vi "XY Graph Delete Consecutive Plots.vi"(8 "Error In":errorcluster, 9 "Plot Indices":i32[](array[numeric]), 11 "XY Graph Ref":refnum<vi>) -> (0 "Error Out":errorcluster, 1 "Plot Names":string[](array[string]), 2 "Graph Caption (or Label)":string, 3 "XY Graph Ref":refnum<vi>)   [LabVIEW 2021, in "XY Graph Add-Ons.lvlib"]
uses:
  XY Graph Add-Ons.lvlib
  Plot Update Steps.ctl
  XY Graph Plot Properties.ctl
  6eef607f-ca58-401d-bd43-5eec63f72193.vi
  XY Graph Get Plots Metadata.vi
  XY Graph Set Plots Metadata.vi
  Graphs.lvlib
  Arrays/Arrays.lvlib
  Error/Error.lvlib
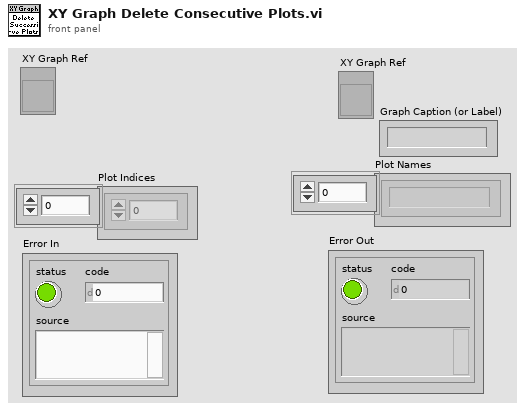
[diagram p1: front panel]
types:
  T1 = typedef "Graphs.lvlib/Plot Update Steps.ctl" = enum16{"Update Plot Styles", "Update Annotation List", "Update Cursor List", "Update Plots", "Quit"}
  T2 = typedef "XY Graph Add-Ons.lvlib/XY Graph Plot Properties.ctl" = cluster{"Plot Index":i32, "Plot.Bar Plot Style":u8, "Plot.DigitalLineStyle":u8, "Plot.TransitionLocation":u8, "Plot.Transition Type":u8, "Plot.Fill To":i16, "Plot.Fill/Pt. Color":u32, "Plot.Label Format":u8, "Plot.Line Style":u8, "Plot.Line Width":u8, "Plot.Plot Color":u32, "Plot.Plot Interpolation":u8, "Plot.Plot Name":string, "Plot.Point Style":u8, "Plot.Visible?":bool, "Plot.XScaleIdx":u32, "Plot.YScaleIdx":u32, "Plot.Anti-aliased":bool}
  T3 = typedef "LVAnnotationListTypeDef.ctl" = cluster{"Name":string, "Color":u32, "Style":u8, "Point Style":u8, "Name Visible":bool, "Allow Drag":bool, "Annotation Mode":u32, "Plot":i32, "Index":i32, "Position":cluster{"X":dbl, "Y":dbl}, "X Scale":u32, "Y Scale":u32, "Show Arrow":bool, "Lock Name":bool, "Plot Area":i32, "Label Offset":cluster{"X":dbl, "Y":dbl}}[]
  T4 = typedef "LVCursorListTypeDef.ctl" = cluster{"Name":string, "Color":u32, "Style":u8, "Point Style":u8, "Name Visible":bool, "Allow Drag":bool, "Cursor Mode":u32, "Plot":i32, "Index":i32, "Position":cluster{"X":dbl, "Y":dbl}, "X Scale":u32, "Y Scale":u32, "Watch Plots":i32[], "Watch All Plots":bool, "Plot Area":i32, "Label Offset":cluster{"X":dbl, "Y":dbl}}[]
  T5 = typedef "XY Graph Add-Ons.lvlib/XY Graph Refnum.ctl" = refnum<vi>
  T6 = cluster{"Name":string, "Color":u32, "Style":u8, "Point Style":u8, "Name Visible":bool, "Allow Drag":bool, "Annotation Mode":u32, "Plot":i32, "Index":i32, "Position":cluster{"X":dbl, "Y":dbl}, "X Scale":u32, "Y Scale":u32, "Show Arrow":bool, "Lock Name":bool, "Plot Area":i32, "Label Offset":cluster{"X":dbl, "Y":dbl}}
  T7 = cluster{"Name":string, "Color":u32, "Style":u8, "Point Style":u8, "Name Visible":bool, "Allow Drag":bool, "Cursor Mode":u32, "Plot":i32, "Index":i32, "Position":cluster{"X":dbl, "Y":dbl}, "X Scale":u32, "Y Scale":u32, "Watch Plots":i32[], "Watch All Plots":bool, "Plot Area":i32, "Label Offset":cluster{"X":dbl, "Y":dbl}}
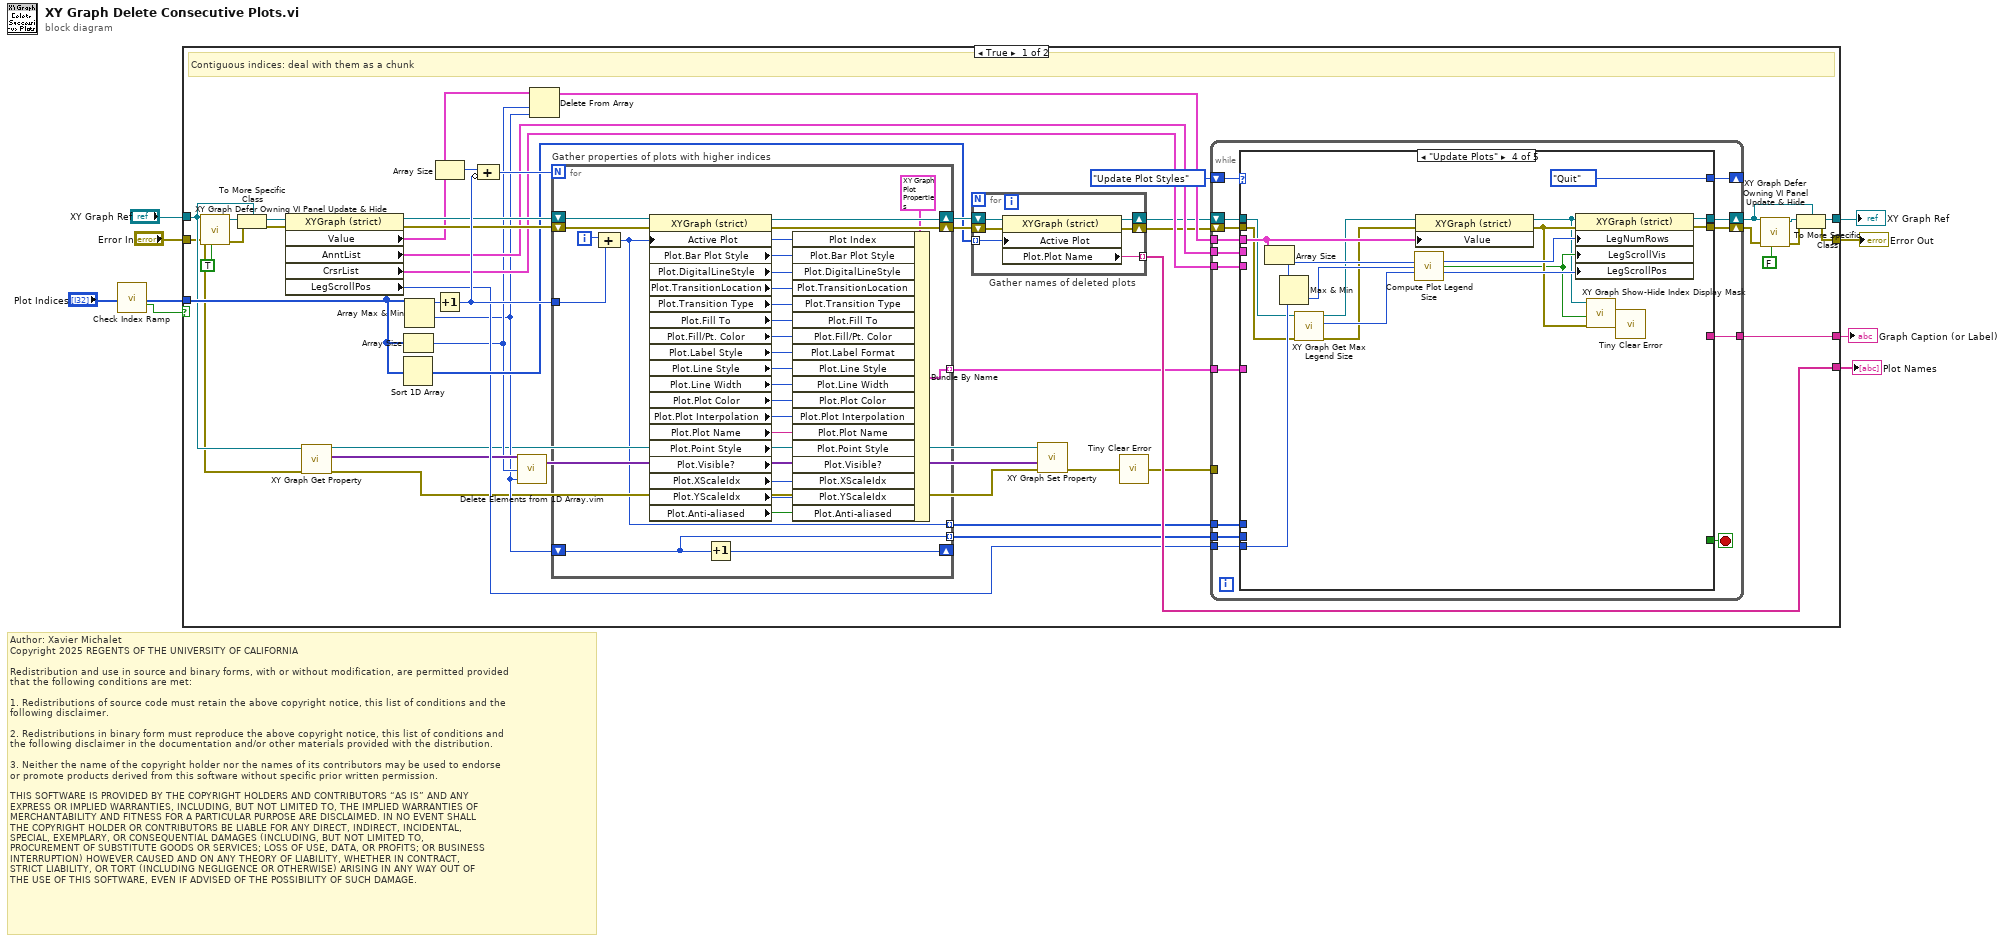
[diagram p0: block diagram]
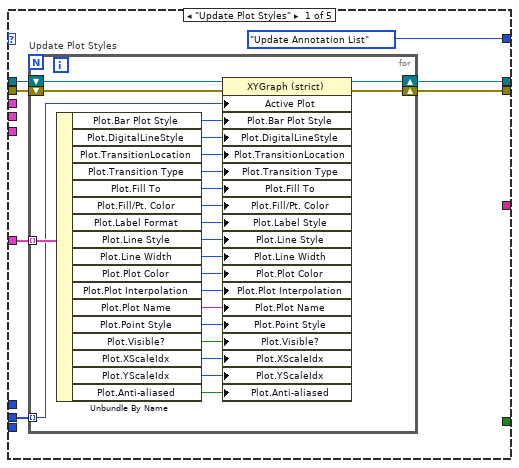
[diagram p2: hidden frame]
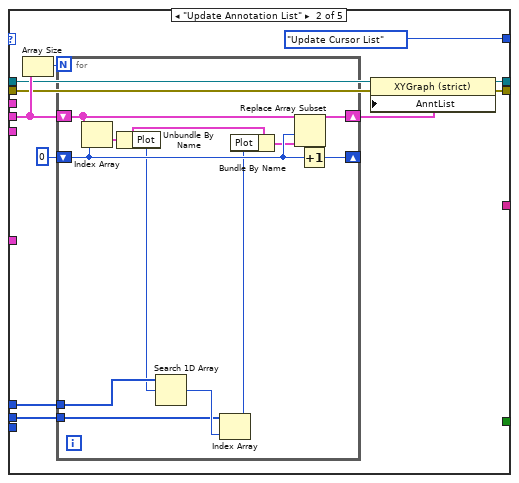
[diagram p3: hidden frame]
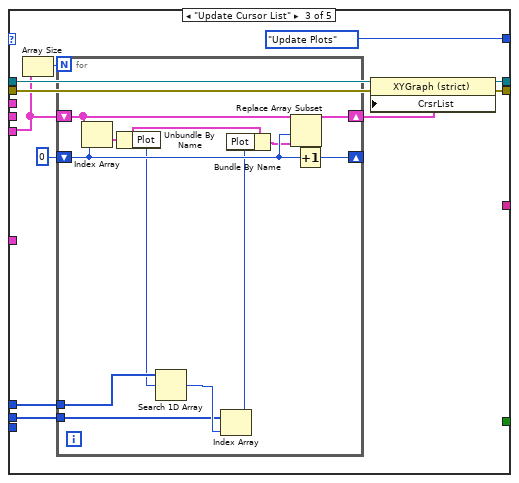
[diagram p4: hidden frame]
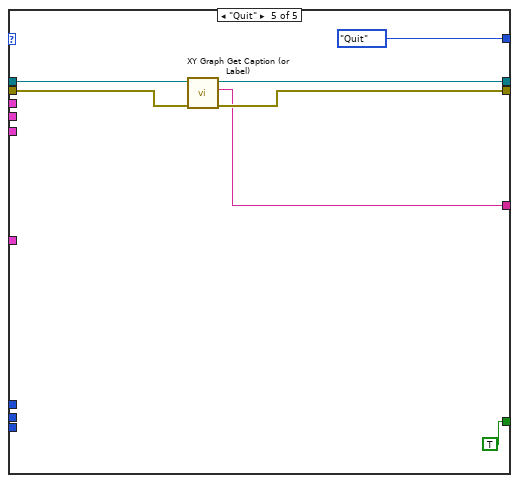
[diagram p5: hidden frame]
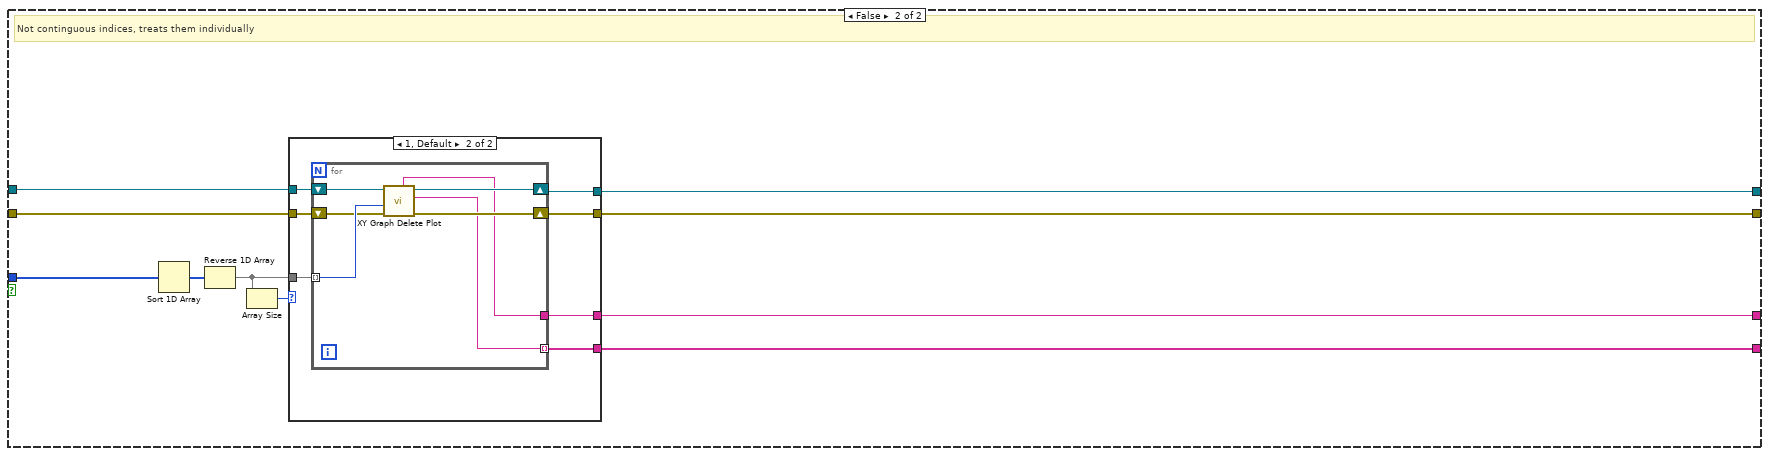
[diagram p6: hidden frame]
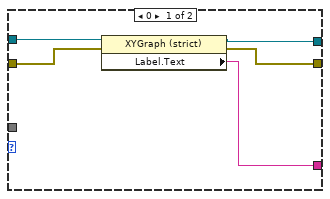
[diagram p7: hidden frame]
diagram:
  # "Author: Xavier Michalet\nCopyright 2025 REGENTS OF THE UNIVERSITY OF CALIFORNIA\n\nRedistribution and use in source and binary forms, with or without modification, are permitted provided\nthat the following conditions are met:\n\n1. Redistributions of source code must retain the above copyright notice, this list of conditions and the\nfollowing disclaimer.\n\n2. Redistributions in binary form must reproduce the above copyright notice, this list of conditions and\nthe following disclaimer in the documentation and/or other materials provided with the distribution.\n\n3. Neither the name of the copyright holder nor the names of its contributors may be used to endorse \nor promote products derived from this software without specific prior written permission.\n\nTHIS SOFTWARE IS PROVIDED BY THE COPYRIGHT HOLDERS AND CONTRIBUTORS “AS IS” AND ANY \nEXPRESS OR IMPLIED WARRANTIES, INCLUDING, BUT NOT LIMITED TO, THE IMPLIED WARRANTIES OF\nMERCHANTABILITY AND FITNESS FOR A PARTICULAR PURPOSE ARE DISCLAIMED. IN NO EVENT SHALL\nTHE COPYRIGHT HOLDER OR CONTRIBUTORS BE LIABLE FOR ANY DIRECT, INDIRECT, INCIDENTAL, \nSPECIAL, EXEMPLARY, OR CONSEQUENTIAL DAMAGES (INCLUDING, BUT NOT LIMITED TO, \nPROCUREMENT OF SUBSTITUTE GOODS OR SERVICES; LOSS OF USE, DATA, OR PROFITS; OR BUSINESS\nINTERRUPTION) HOWEVER CAUSED AND ON ANY THEORY OF LIABILITY, WHETHER IN CONTRACT, \nSTRICT LIABILITY, OR TORT (INCLUDING NEGLIGENCE OR OTHERWISE) ARISING IN ANY WAY OUT OF\nTHE USE OF THIS SOFTWARE, EVEN IF ADVISED OF THE POSSIBILITY OF SUCH DAMAGE."
  n1 = call "Check Index Ramp.vi"("Plot Indices"="Plot Indices") -> ("Plot Indices (dup)"=w1:i32[], "Contiguous?"=w2:bool)  [unwired: 16 in, 1 out]
  n2 = case shown="True" w2 {
    tunnel: "XY Graph Ref" -> [w19 w210]
    tunnel: [w23 w209] -> w8
    tunnel: "Error In" -> [w18 w208]
    tunnel: [w20 w207] -> w6
    tunnel: [w39 w206] -> w5
    tunnel: [w40 w205] -> w4
    tunnel: w1 -> [w46 w212]
    frame True {
      # "Contiguous indices: deal with them as a chunk"
      n3 = call "XY Graph Defer Owning VI Panel Update & Hide.vi"("Defer Owning Panel Update"=TRUE, "error in (no error)"=w18, "XY Graph Refnum in"=w19) -> ("error out"=w24:errorcluster, "XY Graph Refnum out"=w28:refnum<vi>)  [unwired: 7 in]
      n4 = To More Specific Class(target class=w19, reference=w28, error in=w24) -> (specific class reference=w26:refnum<vi>, error out=w25:errorcluster)
      n5 = property class="XYGraph (strict)"(reference=w26, error in=w25) -> (reference out=w49:refnum<vi>, error out=w48:errorcluster, "Value"=w47:cluster{dbl[], dbl[]}[], "AnntList"=w42:T3, "CrsrList"=w41:T4, "LegScrollPos"=w34:u32)
      n6 = call-poly "XY Graph Get Property.vi"("Error In"=w18, "XYGraph Ref"=w19) -> ("Error Out"=w14:errorcluster, "Plot Metadata"=w17:variant[], "XYGraph Ref (dup)"=w10:T5)  [unwired: 6 in, 1 out]
      n7 = Sort 1D Array(array=w46) -> (sorted array=w35:i32[])
      n8 = Array Size(array=w46) -> (size(s)=w16:i32)
      n9 = Array Max & Min(array=w46) -> (max value=w51:i32, min value=w15:i32)  [unwired: 2 out]
      n10 = Array Size(array=w47) -> (size(s)=w54:i32)
      n11 = Increment(x=w51) -> (x+1=w50:i32)
      n12 = Compound Arithmetic op=ADD(w54, invert w50) -> (w52:i32)
      n13 = call "Delete Elements from 1D Array.vim"("index (last elem)"=w15, "length (1)"=w16, "Array"=w17) -> ("array w/ subset deleted"=w11:variant[])  [unwired: 1 out]
      n14 = Delete From Array(array=w47, length=w16, index=w15) -> (array with subset deleted=w45:cluster{dbl[], dbl[]}[])  [unwired: 1 out]
      n15 = for "Gather properties of plots with higher indices" {
        N: w52 -> [_]
        shift-right: [w192] -> w43
        shift-left: w48 -> [w193]
        shift-right: [w194] -> w44
        shift-left: w49 -> [w196]
        tunnel: w50 -> [w174]
        shift-right: [w173] -> _
        shift-left: w15 -> [w172]
        tunnel: [w172] -> w38 mode=indexing
        tunnel: [w171] -> w37 mode=indexing
        tunnel: [w170] -> w36 mode=indexing
        i -> [w195]
        n16 = Compound Arithmetic op=ADD(w195, w174) -> (w170:i32)
        n17 = property class="XYGraph (strict)"(reference=w196, error in=w193, "Active Plot"=w170) -> (reference out=w194:refnum<vi>, error out=w192:errorcluster, "Plot.Bar Plot Style"=w191:u8, "Plot.DigitalLineStyle"=w190:u8, "Plot.TransitionLocation"=w189:u8, "Plot.Transition Type"=w188:u8, "Plot.Fill To"=w187:i16, "Plot.Fill/Pt. Color"=w186:u32, "Plot.Label Style"=w185:u8, "Plot.Line Style"=w184:u8, "Plot.Line Width"=w183:u8, "Plot.Plot Color"=w182:u32, "Plot.Plot Interpolation"=w181:u8, "Plot.Plot Name"=w180:string, "Plot.Point Style"=w179:u8, "Plot.Visible?"=w178:bool, "Plot.XScaleIdx"=w177:u32, "Plot.YScaleIdx"=w176:u32, "Plot.Anti-aliased"=w169:bool)
        n18 = Increment(x=w172) -> (x+1=w173:i32)
        n19 = Bundle By Name(cluster=T2 {"Plot Index"=0, "Plot.Bar Plot Style"=0, "Plot.DigitalLineStyle"=0, "Plot.TransitionLocation"=0, "Plot.Transition Type"=0, "Plot.Fill To"=0, "Plot.Fill/Pt. Color"=0, "Plot.Label Format"=0, "Plot.Line Style"=0, "Plot.Line Width"=0, "Plot.Plot Color"=0, "Plot.Plot Interpolation"=0, "Plot.Plot Name"="", "Plot.Point Style"=0, "Plot.Visible?"=FALSE, "Plot.XScaleIdx"=0, "Plot.YScaleIdx"=0, "Plot.Anti-aliased"=FALSE}, "Plot Index"=w170, "Plot.Bar Plot Style"=w191, "Plot.DigitalLineStyle"=w190, "Plot.TransitionLocation"=w189, "Plot.Transition Type"=w188, "Plot.Fill To"=w187, "Plot.Fill/Pt. Color"=w186, "Plot.Label Format"=w185, "Plot.Line Style"=w184, "Plot.Line Width"=w183, "Plot.Plot Color"=w182, "Plot.Plot Interpolation"=w181, "Plot.Plot Name"=w180, "Plot.Point Style"=w179, "Plot.Visible?"=w178, "Plot.XScaleIdx"=w177, "Plot.YScaleIdx"=w176, "Plot.Anti-aliased"=w169) -> (w171:T2)
      }
      n20 = for "Gather names of deleted plots" {
        shift-right: [w199] -> w32
        shift-left: w43 -> [w200]
        shift-right: [w201] -> w33
        shift-left: w44 -> [w202]
        tunnel: w35 -> [w198] mode=indexing
        tunnel: [w197] -> w40 mode=indexing
        n21 = property class="XYGraph (strict)"(reference=w202, error in=w200, "Active Plot"=w198) -> (reference out=w201:refnum<vi>, error out=w199:errorcluster, "Plot.Plot Name"=w197:string)
      }
      n22 = call-poly "XY Graph Set Property.vi"("error in (no error)"=w14, "Plots Metadata"=w11, "XY Graph Refnum"=w10) -> ("error out"=w13:errorcluster)  [unwired: 7 in, 1 out]
      n23 = call "Tiny Clear Error.vi"("Error In"=w13) -> ("no Error Out"=w12:errorcluster)  [unwired: 8 in]
      n24 = while {
        shift-right: [w64] -> _
        shift-left: Plot_Update_Steps."Update Plot Styles" -> [w66]
        shift-right: [w60] -> w31
        shift-left: w32 -> [w68]
        tunnel: w42 -> [w63]
        tunnel: w45 -> [w62]
        tunnel: w41 -> [w61]
        shift-right: [w67] -> w22
        shift-left: w33 -> [w69]
        tunnel: [w59] -> w39
        tunnel: w38 -> [w58]
        tunnel: w37 -> [w57]
        tunnel: w36 -> [w56]
        tunnel: w34 -> [w55]
        tunnel: w12 -> [_]
        stop <- w65 stop-if-true
        n25 = case shown="\"Update Plots\"" w66 {
          tunnel: w69 -> [w76 w106 w128 w150 w166]
          tunnel: w68 -> [w75 w104 w126 w151 w164]
          tunnel: [w74 w103 w125 w158 w163] -> w60
          tunnel: [w73 w105 w127 w159 w165] -> w67
          tunnel: w58 -> [w70 w101 w131 _ _]
          tunnel: [_ _ _ _ TRUE] -> w65
          tunnel: [Plot_Update_Steps."Update Annotation List" Plot_Update_Steps."Update Cursor List" Plot_Update_Steps."Update Plots" Plot_Update_Steps."Quit" Plot_Update_Steps."Quit"] -> w64
          tunnel: w63 -> [_ w109 _ _ _]
          tunnel: w62 -> [_ _ _ w160 _]
          tunnel: w61 -> [_ _ w123 _ _]
          tunnel: [_ _ _ _ w162] -> w59
          tunnel: w57 -> [w71 _ _ _ _]
          tunnel: w56 -> [_ w100 w122 _ _]
          tunnel: w55 -> [_ _ _ w156 _]
          frame "Update Plot Styles" {
            n26 = for "Update Plot Styles" {
              tunnel: w71 -> [w99] mode=indexing
              shift-right: [w95] -> w74
              shift-left: w75 -> [w96]
              shift-right: [w97] -> w73
              shift-left: w76 -> [w98]
              tunnel: w70 -> [w78] mode=indexing
              n27 = Unbundle By Name(w99) -> ("Plot.Bar Plot Style"=w94:u8, "Plot.DigitalLineStyle"=w93:u8, "Plot.TransitionLocation"=w92:u8, "Plot.Transition Type"=w91:u8, "Plot.Fill To"=w90:i16, "Plot.Fill/Pt. Color"=w89:u32, "Plot.Label Format"=w88:u8, "Plot.Line Style"=w87:u8, "Plot.Line Width"=w86:u8, "Plot.Plot Color"=w85:u32, "Plot.Plot Interpolation"=w84:u8, "Plot.Plot Name"=w83:string, "Plot.Point Style"=w82:u8, "Plot.Visible?"=w81:bool, "Plot.XScaleIdx"=w80:u32, "Plot.YScaleIdx"=w79:u32, "Plot.Anti-aliased"=w77:bool)
              n28 = property class="XYGraph (strict)"(reference=w98, error in=w96, "Active Plot"=w78, "Plot.Bar Plot Style"=w94, "Plot.DigitalLineStyle"=w93, "Plot.TransitionLocation"=w92, "Plot.Transition Type"=w91, "Plot.Fill To"=w90, "Plot.Fill/Pt. Color"=w89, "Plot.Label Style"=w88, "Plot.Line Style"=w87, "Plot.Line Width"=w86, "Plot.Plot Color"=w85, "Plot.Plot Interpolation"=w84, "Plot.Plot Name"=w83, "Plot.Point Style"=w82, "Plot.Visible?"=w81, "Plot.XScaleIdx"=w80, "Plot.YScaleIdx"=w79, "Plot.Anti-aliased"=w77) -> (reference out=w97:T5, error out=w95:errorcluster)
            }
          }
          frame "Update Annotation List" {
            n29 = Array Size(array=w109) -> (size(s)=w108:i32)
            n30 = for {
              N: w108 -> [_]
              shift-right: [w118] -> w102
              shift-left: w109 -> [w120]
              shift-right: [w117] -> _
              shift-left: 0 -> [w119]
              tunnel: w101 -> [w113]
              tunnel: w100 -> [w116]
              n31 = Index Array(array=w120, index=w119) -> (element=w121:T6)
              n32 = Unbundle By Name(w121) -> ("Plot"=w115:i32)
              n33 = Search 1D Array(1D array=w116, element=w115) -> (index of element=w114:i32)  [unwired: 1 in]
              n34 = Index Array(array=w113, index=w114) -> (element=w111:i32)
              n35 = Bundle By Name(cluster=w121, "Plot"=w111) -> (w112:T6)
              n36 = Replace Array Subset(array=w120, new element=w112, index=w119) -> (w118:T3)
              n37 = Increment(x=w119) -> (x+1=w117:i32)
            }
            n38 = property class="XYGraph (strict)"(reference=w106, error in=w104, "AnntList"=w102) -> (reference out=w105:T5, error out=w103:errorcluster)
          }
          frame "Update Cursor List" {
            n39 = Array Size(array=w123) -> (size(s)=w130:i32)
            n40 = for {
              N: w130 -> [_]
              tunnel: w131 -> [w135]
              shift-right: [w140] -> w124
              shift-left: w123 -> [w142]
              shift-right: [w139] -> _
              shift-left: 0 -> [w141]
              tunnel: w122 -> [w138]
              n41 = Index Array(array=w142, index=w141) -> (element=w143:T7)
              n42 = Unbundle By Name(w143) -> ("Plot"=w137:i32)
              n43 = Search 1D Array(1D array=w138, element=w137) -> (index of element=w136:i32)  [unwired: 1 in]
              n44 = Index Array(array=w135, index=w136) -> (element=w133:i32)
              n45 = Bundle By Name(cluster=w143, "Plot"=w133) -> (w134:T7)
              n46 = Replace Array Subset(array=w142, new element=w134, index=w141) -> (w140:T4)
              n47 = Increment(x=w141) -> (x+1=w139:i32)
            }
            n48 = property class="XYGraph (strict)"(reference=w128, error in=w126, "CrsrList"=w124) -> (reference out=w127:T5, error out=w125:errorcluster)
          }
          frame "Update Plots" {
            n49 = Array Size(array=w160) -> (size(s)=w157:i32)
            n50 = Max & Min(x=w157, y=w156) -> (min(x,y)=w155:u32)  [unwired: 1 out]
            n51 = call "XY Graph Get Max Legend Size.vi"("Error In"=w151, "XYGraph Refnum"=w150) -> ("Error Out"=w148:errorcluster, "Max Legend Size"=w152:i32, "XYGraph Refnum"=w149:T5)  [unwired: 6 in, 1 out]
            n52 = call "Compute Plot Legend Size.vi"("# Plots"=w157, "Current Plot (Last)"=w155, "Max Legend Size"=w152) -> ("LegNumRows"=w154:u32, "LegScrollVis"=w145:bool, "LegScrollPos"=w153:u32)  [unwired: 10 in]
            n53 = property class="XYGraph (strict)"(reference=w149, error in=w148, "Value"=w160) -> (reference out=w144:T5, error out=w146:errorcluster)
            n54 = property class="XYGraph (strict)"(reference=w144, error in=w146, "LegNumRows"=w154, "LegScrollVis"=w145, "LegScrollPos"=w153) -> (reference out=w159:T5, error out=w158:errorcluster)
            n55 = call "XY Graph Show-Hide Index Display Mask.vi"("error in (no error)"=w146, "Show(T)/Hide(F)"=w145, "XYGraph Ref"=w144) -> ("error out"=w147:errorcluster)  [unwired: 7 in, 1 out]
            n56 = call "Tiny Clear Error.vi"("Error In"=w147) -> ()  [unwired: 8 in, 1 out]
          }
          frame "Quit" {
            n57 = call "XY Graph Get Caption (or Label).vi"("error in (no error)"=w164, "XY Graph in"=w166) -> ("error out"=w163:errorcluster, "Caption (or Label) Text"=w162:string, "XY Graph out"=w165:T5)  [unwired: 7 in]
          }
        }
      }
      n58 = call "XY Graph Defer Owning VI Panel Update & Hide.vi"("Defer Owning Panel Update"=FALSE, "error in (no error)"=w31, "XY Graph Refnum in"=w22) -> ("error out"=w21:errorcluster, "XY Graph Refnum out"=w30:refnum<vi>)  [unwired: 7 in]
      n59 = To More Specific Class(target class=w22, reference=w30, error in=w21) -> (specific class reference=w23:T5, error out=w20:errorcluster)
    }
    frame False {
      # "Not continguous indices, treats them individually"
      n60 = Sort 1D Array(array=w212) -> (sorted array=w211:i32[])
      n61 = Reverse 1D Array(array=w211) -> (reversed array=w204:i32[])
      n62 = Array Size(array=w204) -> (size(s)=w203:i32)
      n63 = case shown="1, Default" w203 {
        tunnel: w210 -> [w217 w224]
        tunnel: [w215 w223] -> w209
        tunnel: w208 -> [w216 w222]
        tunnel: [w214 w221] -> w207
        tunnel: [w213 w220] -> w206
        tunnel: [_ w219] -> w205
        tunnel: w204 -> [_ w218]
        frame 0 {
          n64 = property class="XYGraph (strict)"(reference=w217, error in=w216) -> (reference out=w215:refnum<vi>, error out=w214:errorcluster, "Label.Text"=w213:string)
        }
        frame 1, Default {
          n65 = for {
            tunnel: w218 -> [w230] mode=indexing
            shift-right: [w227] -> w221
            shift-left: w222 -> [w228]
            tunnel: [w226] -> w220
            tunnel: [w225] -> w219 mode=indexing
            shift-right: [w229] -> w223
            shift-left: w224 -> [w231]
            n66 = call "XY Graph Delete Plot.vi"("Error In"=w228, "Plot Index"=w230, "XYGraph Ref"=w231) -> ("Error Out"=w227:errorcluster, "Plot Name"=w225:string, "XYGraph Ref"=w229:T5, "Graph Caption (or Label)"=w226:string)  [unwired: 5 in]
          }
        }
      }
    }
  }
  "XY Graph Ref" <- w8
  "Error Out" <- w6
  "Graph Caption (or Label)" <- w5
  "Plot Names" <- w4
